vi "Dependency Get Supported Target.vi"(8 "error in (no error)":errorcluster, 11 "Dependency Node in":refnum<k20>) -> (0 "error out":errorcluster, 2 "Supported Target outs":string, 3 "Dependency Node out":refnum<k20>)   [LabVIEW 2019, in "LVLIBP CD XML Updater.lvlib" / "Project XML Editor.lvclass"]
uses:
  Project XML Editor.lvclass
  <vilib>/xml/Close Reference(Node).vi
  <vilib>/xml/NI_XML.lvlib
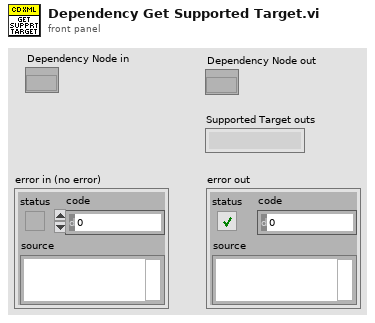
[diagram p1: front panel]
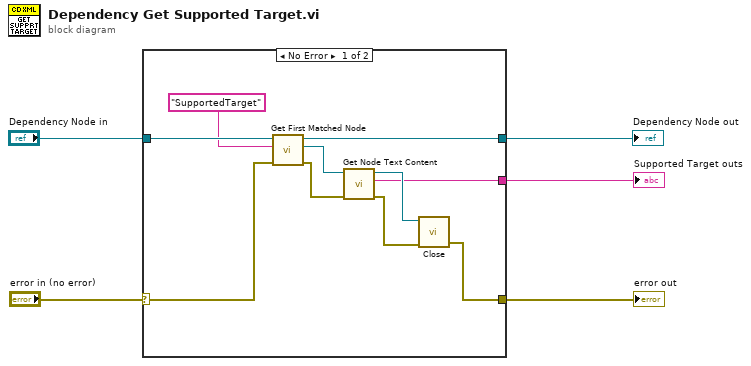
[diagram p0: block diagram]
diagram:
  n1 = case shown="No Error" "error in (no error)" {
    selector: "error in (no error)" -> [w8 w17]
    tunnel: "Dependency Node in" -> [w14 w16]
    tunnel: [w9 _] -> w4
    tunnel: [w7 w17] -> w2
    tunnel: [w6 w16] -> w1
    frame No Error {
      n2 = call <vilib>:"Get First Matched Node.vi"("error in (no error)"=w8, "XPath expression"="SupportedTarget", "node in"=w14) -> ("error out"=w15:errorcluster, "node result"=w12:refnum<k20>, "node out"=w6:refnum<k20>)  [unwired: 6 in]
      n3 = call <vilib>:"Get Node Text Content.vi"("error in (no error)"=w15, "node in"=w12) -> ("error out"=w10:errorcluster, "node text"=w9:string, "node out"=w13:refnum<k20>)  [unwired: 7 in]
      n4 = call-poly <vilib>:"Close.vi"("error in (no error)"=w10, "node"=w13) -> ("error out"=w7:errorcluster)  [unwired: 7 in]
    }
    frame Error {
    }
  }
  "Supported Target outs" <- w4
  "error out" <- w2
  "Dependency Node out" <- w1
